vi "TRIG_CHAN_ROUT_READ.vi"(0 "VISA IN":refnum<visa-resource-name>, 1 "Ready":string(combo)="MAIN", 5 "error in":errorcluster, 7 "Channel":i32) -> (14 "VISA Out":refnum<visa-resource-name>, 19 "error out":errorcluster)   [LabVIEW 2018, in "PNA-X.lvlib"]
doc: "TRIGger:CHANnel<ch>:ROUTe:READy <char> \n(Read-Write) Specifies the connector to use for the external trigger OUT ready line. \nParameters \n<ch> Any existing channel number. If unspecified, value is set to 1. \n<char> Choose from: \nMAIN - Meas trig ready \nMATH - Material handler pin 21 \nAUXT - AUX I/O pin 18 (PNA-L and E836xB ONLY) \nExamples TRIG:CHAN:ROUT:READ main \ntrigger:channel2:route:ready auxt \nQuery Syntax TRIGger:CHANnel<ch>:ROUTe:READy? \nReturn Type Character \nDefault \n1894"
uses:
  PNA-X.lvlib
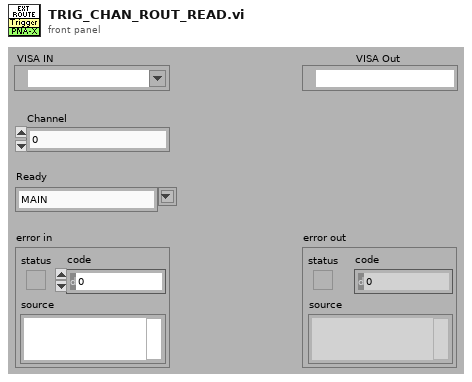
[diagram p1: front panel]
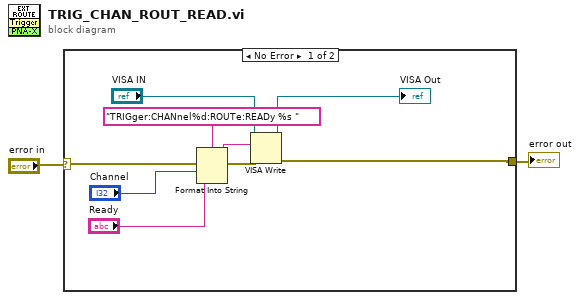
[diagram p0: block diagram]
diagram:
  n1 = case shown="No Error" "error in" {
    selector: "error in" -> [w11 w12]
    tunnel: [w6 w12] -> w1
    frame No Error {
      n2 = Format Into String(format string="TRIGger:CHANnel%d:ROUTe:READy %s " ("Cmdline"), error in=w11, "Channel", "Ready") -> (resulting string=w9:string, error out=w10:errorcluster)  [unwired: 1 in]
      n3 = VISA Write(VISA resource name="VISA IN", write buffer=w9, error in (no error)=w10) -> (VISA resource name out=→"VISA Out":refnum<visa-resource-name>, error out=w6:errorcluster)  [unwired: 1 out]
    }
    frame Error {
    }
  }
  "error out" <- w1
